vi "Initialize.vi"(8 "error in (no error)":errorcluster, 10 "Laser Configuration":T1, 11 "Cobolt in":refnum<class "Cobolt Laser.lvclass">) -> (0 "error out":errorcluster, 3 "Cobolt out":refnum<class "Cobolt Laser.lvclass">)   [LabVIEW 2023, in "Cobolt Laser.lvlib" / "Cobolt Laser.lvclass"]
uses:
  Cobolt Laser.lvclass
  Resources/Type Defs/Laser Configuration.ctl
  Cobolt Laser.lvclass/Cobolt Laser.ctl
  <vilib>/Instr/_visa.llb/VISA Configure Serial Port (Instr).vi
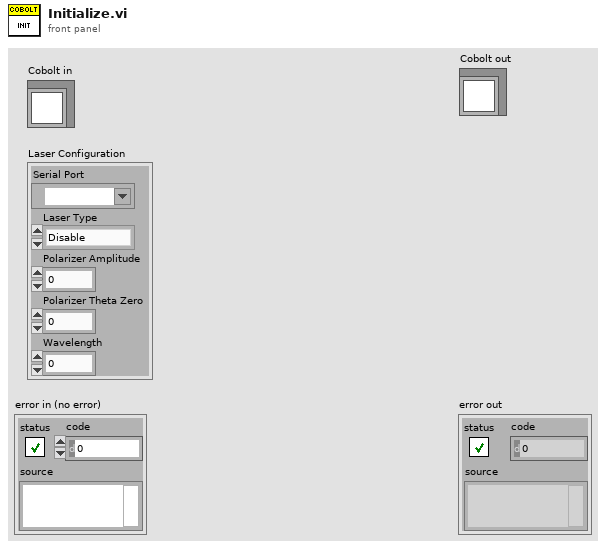
[diagram p1: front panel]
types:
  T1 = typedef "Laser Configuration.ctl" = cluster{"Serial Port":refnum<visa-resource-name>, "Laser Type":enum16{"Disable", "Laser Quantum", "Coherent OBIS", "PRM1-Z8", "Coherent HOPS", "Cobolt"}, "Polarizer Amplitude":dbl, "Polarizer Theta Zero":dbl, "Wavelength":u16}
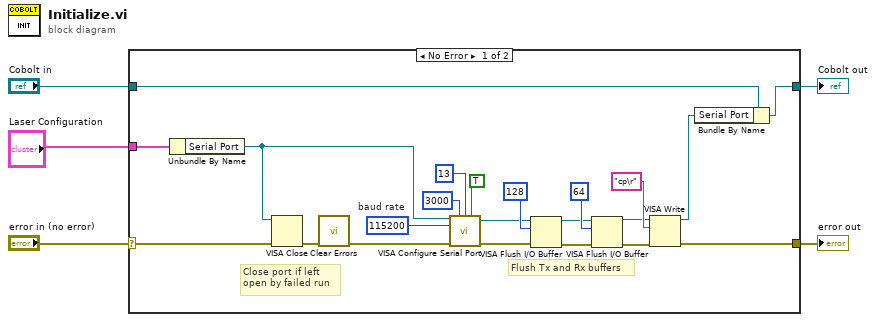
[diagram p0: block diagram]
diagram:
  n1 = case shown="No Error" "error in (no error)" {
    selector: "error in (no error)" -> [w20 w28]
    tunnel: [w7 w28] -> w4
    tunnel: "Laser Configuration" -> [w17 _]
    tunnel: "Cobolt in" -> [w19 w29]
    tunnel: [w18 w29] -> w1
    frame No Error {
      w26 = u32 115200  # baud rate
      # "Flush Tx and Rx buffers"
      # "Close port if left\nopen by failed run"
      n2 = Unbundle By Name(w17) -> ("Serial Port"=w22:refnum<visa-resource-name>)
      n3 = VISA Close(VISA resource name=w22, error in (no error)=w20) -> (error out=w24:errorcluster)
      n4 = call <vilib>:"Clear Errors.vi"("error in (no error)"=w24) -> ("error out"=w23:errorcluster)  [unwired: 5 in, 1 out]
      n5 = call-poly "VISA Configure Serial Port"("VISA resource name"=w22, "timeout (10sec)"=u32 3000, "termination char\n(0xA = '\\n' = LF)"=u8 13 ("termination char\n(0xA = '\\n' = LF)"), "Enable Termination\nChar (T)"=TRUE ("Enable Termination\nChar (T)"), "baud rate (9600)"=w26, "error in (no error)"=w23) -> ("VISA resource name out"=w10:refnum<visa-resource-name>, "error out"=w11:errorcluster)  [unwired: 8 in]
      n6 = VISA Flush I/O Buffer(VISA resource name=w10, mask (16)=u16 128, error in (no error)=w11) -> (VISA resource name out=w13:refnum<visa-resource-name>, error out=w12:errorcluster)
      n7 = VISA Flush I/O Buffer(VISA resource name=w13, mask (16)=u16 64, error in (no error)=w12) -> (VISA resource name out=w8:refnum<visa-resource-name>, error out=w9:errorcluster)
      n8 = VISA Write(VISA resource name=w8, write buffer="cp\r", error in (no error)=w9) -> (VISA resource name out=w6:refnum<visa-resource-name>, error out=w7:errorcluster)  [unwired: 1 out]
      n9 = Bundle By Name(cluster=w19, "Serial Port"=w6) -> (w18:refnum<class "Cobolt Laser.lvclass">)
    }
    frame Error {
    }
  }
  "error out" <- w4
  "Cobolt out" <- w1
